vi "Abadines_ClientA.vi"   [LabVIEW 2013]
uses:
  <vilib>/NXT/Block Support/NXT_MessageMailbox.ctl
  <vilib>/NXT/Block Support/NXT_OutputPort.ctl
  <vilib>/NXT/NXTIO Xnodes/NXTIONodeSubVIs/NXTStopMotors.vi
  <vilib>/NXT/NXTIO Xnodes/AddressXNode/NXTIOAddress.xnode
  <vilib>/NXT/NXTIO Xnodes/NXTIOXNode/NXTIO.xnode
  <vilib>/NXT/Subs/LVHSConnector.ctl
  <vilib>/NXT/LegoClasses/BrickReference/BrickReference.lvclass
types:
  T1 = typedef "LVHSConnector.ctl" = refnum<class "BrickReference.lvclass">
  T2 = typedef "NXT_OutputPort.ctl" = u8
  T3 = typedef "NXT_MessageMailbox.ctl" = u8
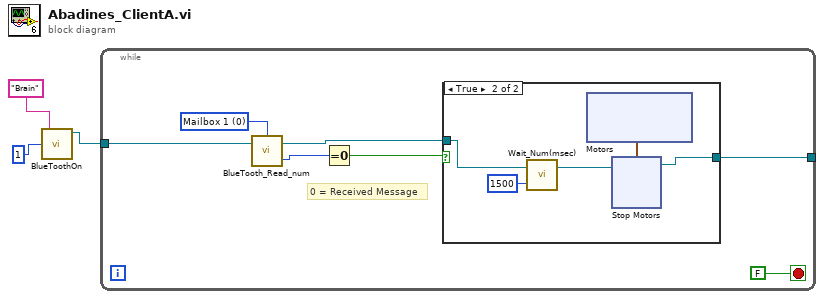
[diagram p0: block diagram]
diagram:
  n1 = call "BlueToothOn.vi"("Connection"=u8 1, "Partner Name"="Brain") -> ("NXT/EV3 2"=w1:T1)  [unwired: 1 in, 3 out]
  n2 = while {
    tunnel: w1 -> [w9]
    tunnel: [w5] -> _
    stop <- FALSE stop-if-true
    w10 = T3 0 items=["Mailbox 1", "Mailbox 2", "Mailbox 3", "Mailbox 4", "Mailbox 5", "Mailbox 6", "Mailbox 7", "Mailbox 8", "Mailbox 9", "Mailbox 10"] ("Mailbox")
    # "0 = Received Message"
    n3 = call <vilib>:"BlueTooth_Read_num.vi"("NXT/EV3"=w9, "Mailbox"=w10) -> ("Message"=w8:i32, "NXT/EV3"=w6:T1)  [unwired: 1 in]
    n4 = Equal To 0?(x=w8) -> (x = 0?=w7:bool)
    n5 = case shown="True" w7 {
      tunnel: w6 -> [w11 w14]
      tunnel: [w11 w15] -> w5
      frame False {
        # "Do Nothing!"
      }
      frame True {
        n6 = call <vilib>:"Wait_Num(msec).vi"("Time (100 msec)"=u32 1500, "NXT/EV3"=w14) -> ("NXT/EV3"=w13:T1)  [unwired: 2 in]
        n7 = xnode "Motors"() -> ("Motor"=w16:cluster{"Port":T2, "Port":T2})
        n8 = xnode "Stop Motors"("Motors"=w16, "NXT/EV3"=w13) -> ("NXT/EV3"=w15:T1)
      }
    }
  }
